vi "Open_Create__Log_File.vi"(0 "File Path Control":path, 5 "Enum":enum16{"CSV File", "Text File"}(ring), 11 "Error In":errorcluster) -> (4 "refnum out":refnum<file>, 6 "File Path":path, 15 "Error Out":errorcluster)   [LabVIEW 2021]
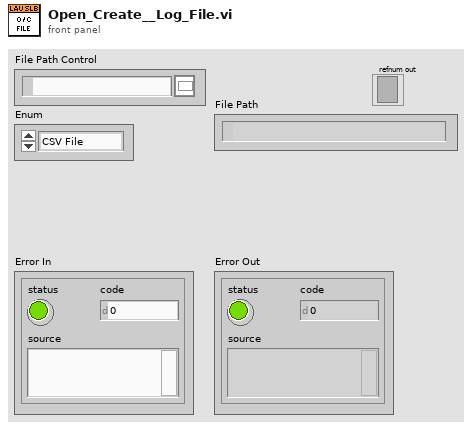
[diagram p1: front panel]
types:
  T1 = enum16{"open", "replace", "create", "open or create", "replace or create", "replace or create with confirmation"}
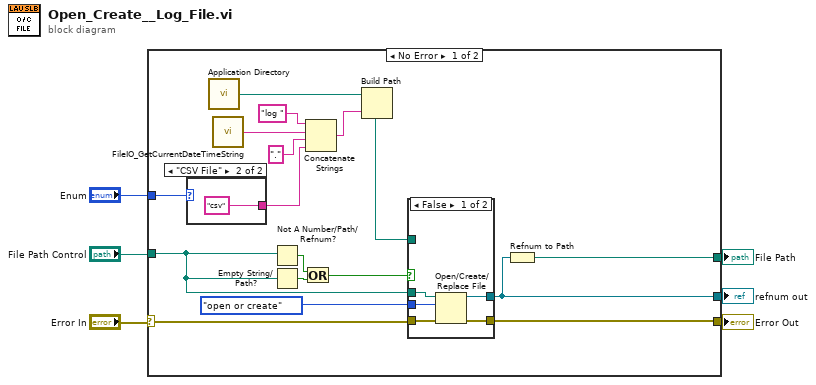
[diagram p0: block diagram]
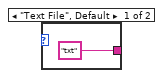
[diagram p2: hidden frame]
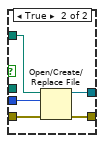
[diagram p3: hidden frame]
diagram:
  n1 = case shown="No Error" "Error In" {
    selector: "Error In" -> [w19 w36]
    tunnel: "File Path Control" -> [w17 _]
    tunnel: [w16 _] -> w5
    tunnel: [w18 w36] -> w3
    tunnel: [w15 _] -> w2
    tunnel: "Enum" -> [w7 _]
    frame No Error {
      n2 = case shown="\"CSV File\"" w7 {
        tunnel: ["txt" "csv"] -> w8
        frame "Text File", Default {
        }
        frame "CSV File" {
        }
      }
      n3 = call <vilib>:"Application Directory.vi"() -> ("Application Directory"=w14:path)
      n4 = call "FileIO_GetCurrentDateTimeString.vi"() -> ("Date/Time String"=w11:string)  [unwired: 14 in, 1 out]
      n5 = Not A Number/Path/Refnum?(number/path/refnum=w17) -> (NaN/Path/Refnum?=w23:bool)
      n6 = Empty String/Path?(string/path=w17) -> (empty?=w22:bool)
      n7 = Or(x=w23, y=w22) -> (x .or. y?=w21:bool)
      n8 = Concatenate Strings("log " ("string"), w11, "." ("string"), w8) -> (w13:string)
      n9 = Build Path(base path=w14, name or relative path=w13) -> (appended path=w10:path)
      n10 = case shown="False" w21 {
        tunnel: T1."open or create" ("operation (0:open)") -> [w28 w35]
        tunnel: [w29 w34] -> w16
        tunnel: w17 -> [w30 _]
        tunnel: w19 -> [w27 w33]
        tunnel: [w26 w32] -> w18
        tunnel: w10 -> [_ w31]
        frame False {
          n11 = Open/Create/Replace File(file path (use dialog)=w30, error in=w27, operation (0:open)=w28) -> (refnum out=w29:refnum<file>, error out=w26:errorcluster)  [unwired: 3 in, 1 out]
        }
        frame True {
          n12 = Open/Create/Replace File(file path (use dialog)=w31, error in=w33, operation (0:open)=w35) -> (refnum out=w34:refnum<file>, error out=w32:errorcluster)  [unwired: 3 in, 1 out]
        }
      }
      n13 = Refnum to Path(1:w16) -> (0:w15:path)
    }
    frame Error {
    }
  }
  "Error Out" <- w3
  "refnum out" <- w5
  "File Path" <- w2
